vi "Set Function Data Analog Out.vi"(6 "cdData":i32=16384, 7 "rgdData":dbl[](array[numeric])=array[16384 elements], 8 "error in (no error)":errorcluster, 9 "node":T1, 10 "idxChannel":i32, 11 "hdwf":i32) -> (0 "error out":errorcluster, 3 "hdwf out":i32)   [LabVIEW 2014, in "AnalogDiscSDKLv.lvlib"]
doc: "extern \"C\" __declspec(dllexport) int SetFunctionData_AnalogOut(\n HDWF hdwf,\n int idxChannel,\n AnalogOutNode node,\n double rgdData[16384], int cdData\n );"
uses:
  <instrlib>/AnalogDiscSDKLv/AnalogDiscSDKLv.lvlib
  <instrlib>/AnalogDiscSDKLv/VIs/DWF_Node.ctl
  <instrlib>/AnalogDiscSDKLv/AnalogDiscSDKLv.dll
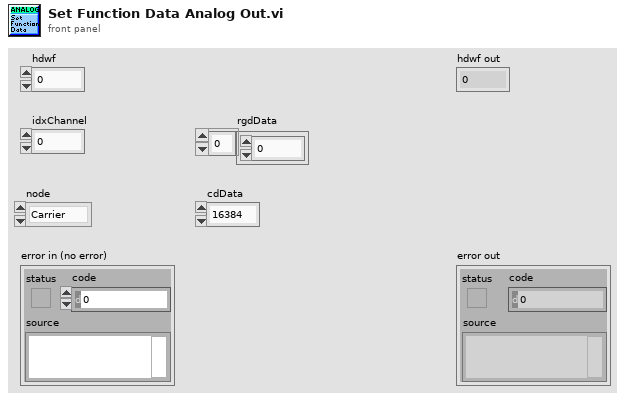
[diagram p1: front panel]
types:
  T1 = typedef "AnalogDiscSDKLv.lvlib/DWF_Node.ctl" = enum16{"Carrier", "FM", "AM"}
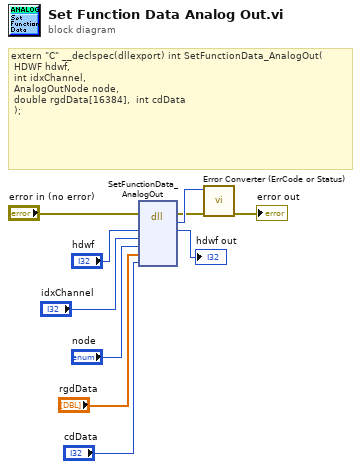
[diagram p0: block diagram]
diagram:
  # "extern \"C\" __declspec(dllexport) int SetFunctionData_AnalogOut(\n\tHDWF hdwf,\n\tint idxChannel,\n\tAnalogOutNode node,\n\tdouble rgdData[16384], \tint cdData\n\t);"
  n1 = dll-call lib="C:/Program Files (x86)/National Instruments/LabVIEW 2014/instr.lib/AnalogDiscSDKLv/AnalogDiscSDKLv.*" fn="SetFunctionData_AnalogOut"(error in="error in (no error)", "hdwf"="hdwf", "idxChannel"="idxChannel", "node"="node", "rgdData"="rgdData", "cdData"="cdData") -> (error out=w2:errorcluster, w3:i32, "hdwf"=→"hdwf out":i32)  [unwired: 6 in, 1 out]
  n2 = call <instrlib>:"Error Converter (ErrCode or Status).vi"("error in (no error)"=w2, "error code"=w3) -> ("error out"=→"error out":errorcluster)  [unwired: 9 in]
